vi "TransferFile - From Data.vi"(5 "ChunkSize (1M)":u32=1000000, 7 "data in":string, 8 "error in (no error)":errorcluster, 9 "Choose the Destination File Folder (Absolute Path) for AWG's files system":path, 10 "Set File Name (with Extension)":string, 11 "VISA resource name":refnum<visa-resource-name>) -> (0 "error out":errorcluster, 3 "VISA resource name out":refnum<visa-resource-name>)   [LabVIEW 2020, in "Active Technologies AWG3000.lvlib"]
doc: "Transfer data string to file in AWG."
uses:
  Active Technologies AWG3000.lvlib
panel:
  # "Note: for the drive C is allowed transfer a file only to the default folder or to its subdirectories. \nNo limitation for the other drives.\nTo know the default folder, run GetDefaultDriveCFolder.vi."
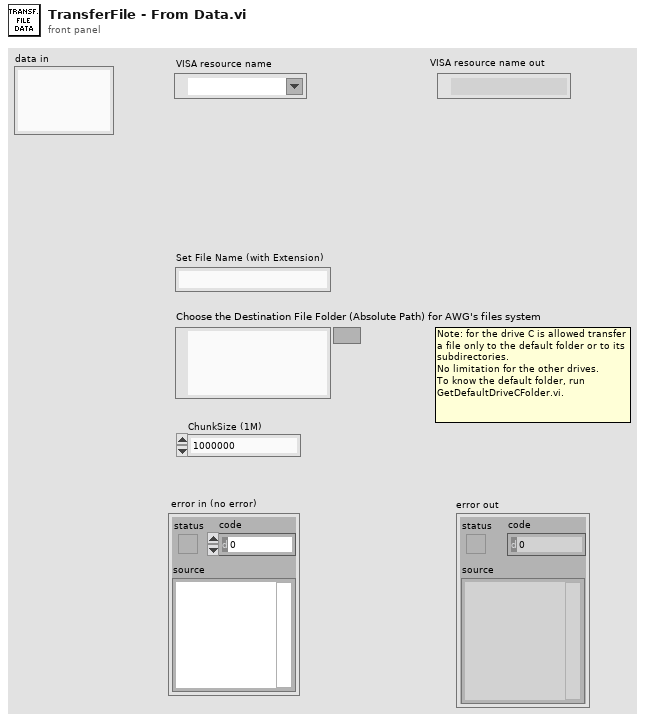
[diagram p1: front panel]
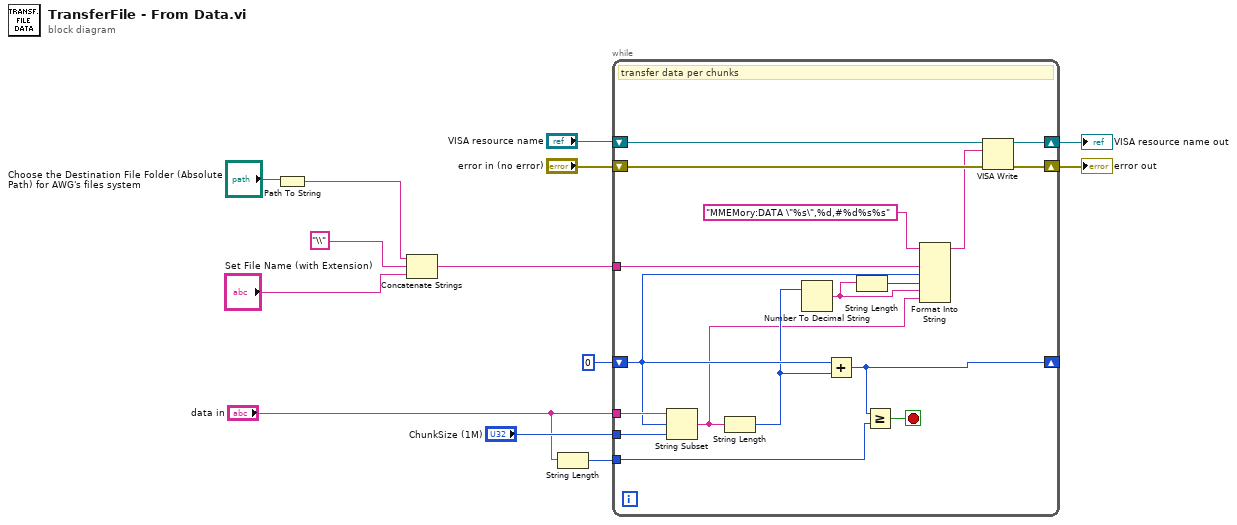
[diagram p0: block diagram]
diagram:
  n1 = Path To String(path="Choose the Destination File Folder (Absolute Path) for AWG's files system") -> (string=w12:string)
  n2 = Concatenate Strings(w12, "\\" ("string"), "Set File Name (with Extension)") -> (w9:string)
  n3 = String Length(string="data in") -> (length=w5:i32)
  n4 = while {
    tunnel: w9 -> [w30]
    shift-right: [w22] -> _
    shift-left: 0 -> [w24]
    tunnel: "data in" -> [w26]
    tunnel: "ChunkSize (1M)" -> [w25]
    tunnel: w5 -> [w21]
    shift-right: [w18] -> w1
    shift-left: "error in (no error)" -> [w17]
    shift-right: [w16] -> w3
    shift-left: "VISA resource name" -> [w15]
    stop <- w20 stop-if-true
    # "transfer data per chunks"
    n5 = String Subset(string=w26, offset (0)=w24, length (rest)=w25) -> (substring=w19:string)
    n6 = String Length(string=w19) -> (length=w23:i32)
    n7 = Number To Decimal String(number=w23) -> (decimal integer string=w27:string)  [unwired: 1 in]
    n8 = Add(x=w24, y=w23) -> (x+y=w22:i32)
    n9 = String Length(string=w27) -> (length=w28:i32)
    n10 = Greater Or Equal?(x=w22, y=w21) -> (x >= y?=w20:bool)
    n11 = Format Into String(format string="MMEMory:DATA \"%s\",%d,#%d%s%s" ("write buffer"), w30, w24, w28, w27, w19) -> (resulting string=w14:string)  [unwired: 2 in, 1 out]
    n12 = VISA Write(VISA resource name=w15, write buffer=w14, error in (no error)=w17) -> (VISA resource name out=w16:refnum<visa-resource-name>, error out=w18:errorcluster)  [unwired: 1 out]
  }
  "VISA resource name out" <- w3
  "error out" <- w1
